vi "Launcher.vi"() -> (0 "error out":errorcluster)   [LabVIEW 2024]
uses:
  Application/Demo.vi
  Application/Main.vi
  Application/Application.lvlib
  Modules/Data Base/DataBase - Top VI.vi
  Modules/Data Base/Data Base.lvlib
  Modules/Error Handler/Error - Top VI.vi
  Modules/Error Handler/Error Handler.lvlib
  Modules/Session Scanner/Scanner - Top VI.vi
  Modules/Session Scanner/Session Scanner.lvlib
  Modules/User Interface/UI - Top VI.vi
  Modules/User Interface/User Interface.lvlib
panel:
  out "error out 2":errorcluster
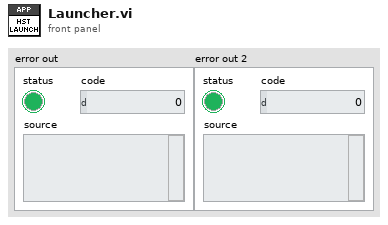
[diagram p1: front panel]
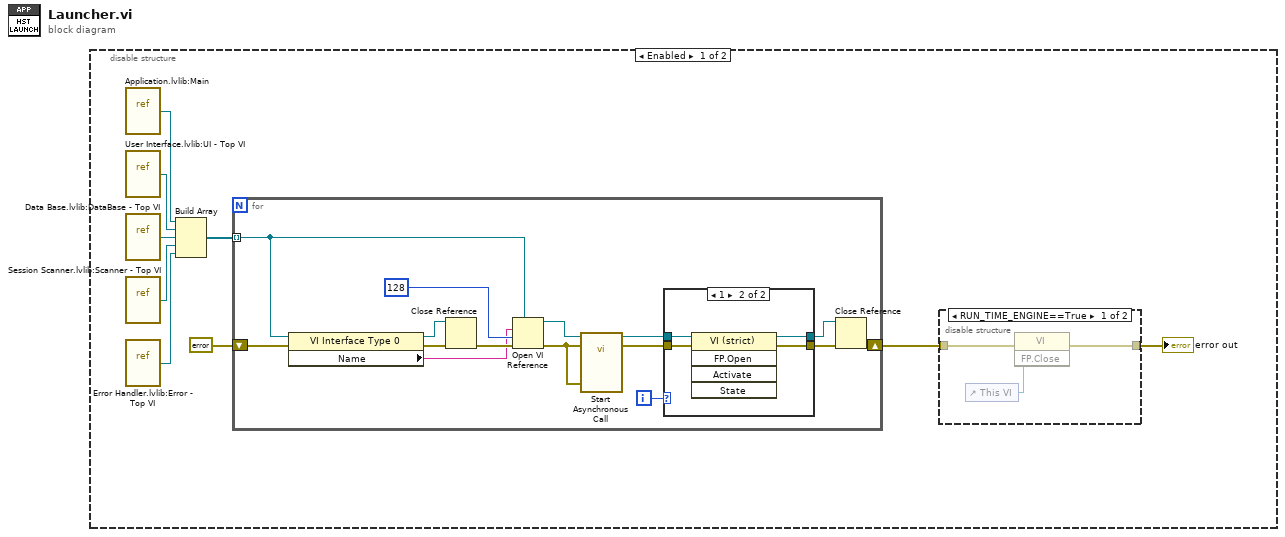
[diagram p0: block diagram]
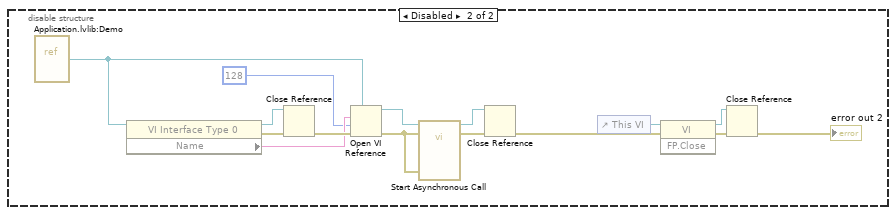
[diagram p4: hidden frame]
diagram:
  n1 = disable-structure shown="Enabled" {
    frame Enabled {
      n2 = vi-ref "Application.lvlib:Main.vi"() -> (w5:refnum<vi>)
      n3 = vi-ref "User Interface.lvlib:UI - Top VI.vi"() -> (w4:refnum<vi>)
      n4 = vi-ref "Data Base.lvlib:DataBase - Top VI.vi"() -> (w3:refnum<vi>)
      n5 = vi-ref "Session Scanner.lvlib:Scanner - Top VI.vi"() -> (w2:refnum<vi>)
      n6 = vi-ref "Error Handler.lvlib:Error - Top VI.vi"() -> (w1:refnum<vi>)
      n7 = Build Array(w5, w4, w3, w2, w1) -> (w6:refnum<vi>[])
      n8 = for {
        shift-right: [w11] -> w8
        shift-left: errorcluster {"status"=FALSE, "code"=0, "source"=""} ("error out") -> [w18]
        tunnel: w6 -> [w17] mode=indexing
        i -> [w20]
        n9 = property class="VI Interface Type 0"(reference=w17, error in=w18) -> (reference out=w15:refnum<vi>, error out=w16:errorcluster, "Name"=w13:string)
        n10 = Close Reference(reference=w15, error in (no error)=w16) -> (error out=w14:errorcluster)
        n11 = Open VI Reference(type specifier VI Refnum (for type only)=w17, vi path=w13, options=128, error in (no error)=w14) -> (vi reference=w19:refnum<vi>, error out=w23:errorcluster)  [unwired: 2 in]
        n12 = call-by-ref "Start Asynchronous Call"(reference=w19, error in=w23, "error in"=w23) -> (reference out=w12:refnum<vi>, error out=w22:errorcluster)  [unwired: 10 in, 1 out]
        n13 = case shown="1" w20 {
          tunnel: w12 -> [w25 w30]
          tunnel: w22 -> [w26 w29]
          tunnel: [w26 w28] -> w21
          tunnel: [w25 w27] -> w10
          frame Default {
          }
          frame 1 {
            n14 = invoke class="VI (strict)" method="FP.Open"(reference=w30, error in=w29) -> (reference out=w27:refnum<vi>, error out=w28:errorcluster)  [unwired: 3 in, 3 out]
          }
        }
        n15 = Close Reference(reference=w10, error in (no error)=w21) -> (error out=w11:errorcluster)
      }
      n16 = disable-structure shown="RUN_TIME_ENGINE==True" {
        disable-tunnel: w8 -> [w33 _]
        disable-tunnel: [w32 _] -> w7
        frame condition #0 {
          n17 = control-ref of="This VI"() -> (w31:refnum<vi>)
          n18 = invoke class="VI" method="FP.Close"(reference=w31, error in=w33) -> (error out=w32:errorcluster)  [unwired: 1 in, 2 out]
        }
        frame condition #1 (active) {
        }
      }
      "error out" <- w7
    }
    frame Disabled {
      n19 = vi-ref "Application.lvlib:Demo.vi"() -> (w39:refnum<vi>)
      n20 = property class="VI Interface Type 0"(reference=w39) -> (reference out=w44:refnum<vi>, error out=w45:errorcluster, "Name"=w42:string)  [unwired: 1 in]
      n21 = Close Reference(reference=w44, error in (no error)=w45) -> (error out=w43:errorcluster)
      n22 = Open VI Reference(type specifier VI Refnum (for type only)=w39, vi path=w42, options=128, error in (no error)=w43) -> (vi reference=w46:refnum<vi>, error out=w48:errorcluster)  [unwired: 2 in]
      n23 = call-by-ref "Start Asynchronous Call"(reference=w46, error in=w48, "error in"=w48) -> (reference out=w41:refnum<vi>, error out=w47:errorcluster)  [unwired: 10 in, 1 out]
      n24 = Close Reference(reference=w41, error in (no error)=w47) -> (error out=w35:errorcluster)
      n25 = control-ref of="This VI"() -> (w36:refnum<vi>)
      n26 = invoke class="VI" method="FP.Close"(reference=w36, error in=w35) -> (reference out=w38:refnum<vi>, error out=w37:errorcluster)  [unwired: 1 in, 1 out]
      n27 = Close Reference(reference=w38, error in (no error)=w37) -> (error out=→"error out 2":errorcluster)
    }
  }
